vi "Read guider queue.vi"(8 "error in (no error)":errorcluster, 11 "GuiderSetup in":refnum<class "GuiderSetup.lvclass">) -> (0 "error out":errorcluster, 2 "guider queue":refnum<queue>, 3 "GuiderSetup out":refnum<class "GuiderSetup.lvclass">)   [LabVIEW 2018, in "GuiderSetup.lvclass"]
uses:
  GuiderSetup.lvclass
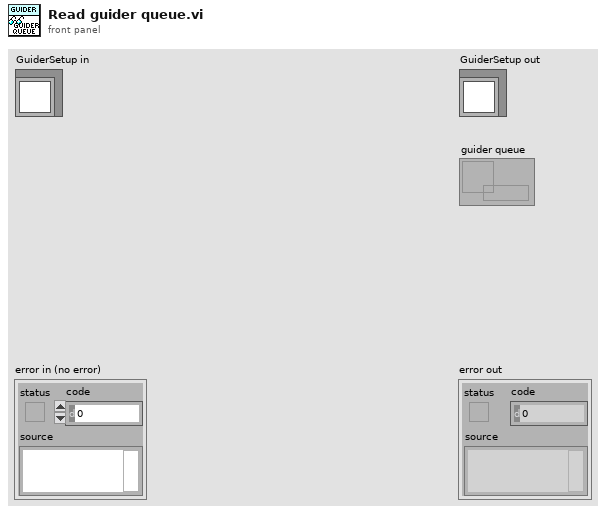
[diagram p1: front panel]
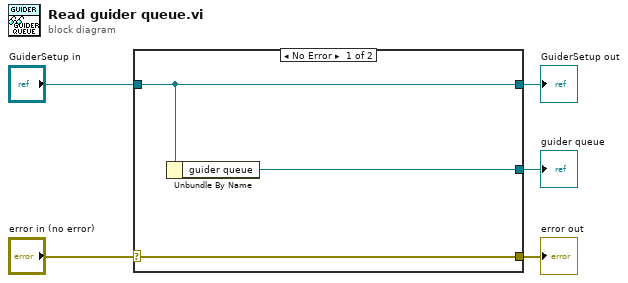
[diagram p0: block diagram]
diagram:
  n1 = case shown="No Error" "error in (no error)" {
    selector: "error in (no error)" -> [w8 w9]
    tunnel: [w8 w9] -> w4
    tunnel: [w7 w10] -> w2
    tunnel: "GuiderSetup in" -> [w7 w10]
    tunnel: [w6 _] -> w1
    frame No Error {
      n2 = Unbundle By Name(w7) -> ("guider queue"=w6:refnum<queue>)
    }
    frame Error {
    }
  }
  "error out" <- w4
  "GuiderSetup out" <- w2
  "guider queue" <- w1
